vi "Encode_SignedRatio.vi"(1 "Signed Ratio":dbl[](array[numeric])) -> (0 "Little Endian":u8[](array[numeric]))   [LabVIEW 2015, in "navX Library v3.lvlib" / "navX Registry Cache.lvclass"]
uses:
  navX Registry Cache.lvclass
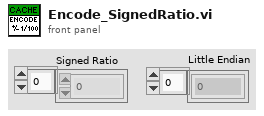
[diagram p1: front panel]
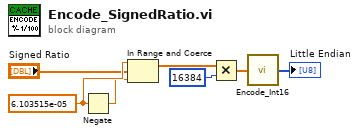
[diagram p0: block diagram]
diagram:
  w6 = 6.103515e-05
  n1 = Negate(x=w6) -> (-x=w3:dbl)
  n2 = In Range and Coerce(upper limit=w6, x="Signed Ratio", lower limit=w3) -> (coerced(x)=w5:dbl[])  [unwired: 1 out]
  n3 = Multiply(x=w5, y=u16 16384) -> (x*y=w2:dbl[])
  n4 = call "Encode_Int16.vi"("Int16"=w2) -> ("Little Endian"=→"Little Endian":u8[])
